vi "LED Lights Subsystem.vi"(8 "error in":errorcluster) -> ()   [LabVIEW 2015]
uses:
  <vilib>/Rock Robotics/SystemInterfaces/i2clib/i2c_bus.ctl
panel:
  in  "Send":bool
  in  "Light ID":u8=3
  in  "Blue":u8=153
  in  "Green":u8=12
  in  "Red":u8=64
  out "error out":errorcluster
  out "open error out":errorcluster
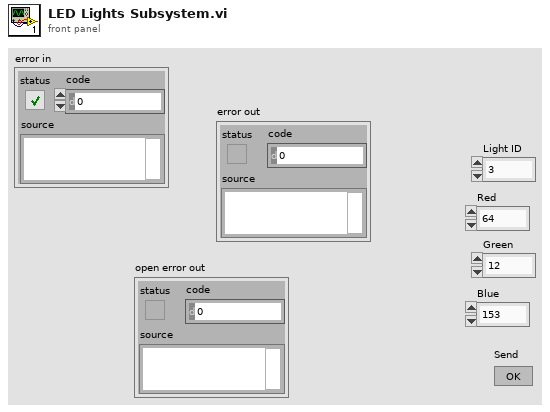
[diagram p1: front panel]
types:
  T1 = typedef "i2c_bus.ctl" = enum16{"I2C On-Board", "I2C MXP", "Invalid"}
  T2 = typedef "WPI_I2CDevRef.ctl" = cluster{"DevStatus":errorcluster, "Device Address":u8, "Handle":i32, "I2C Bus":T1}
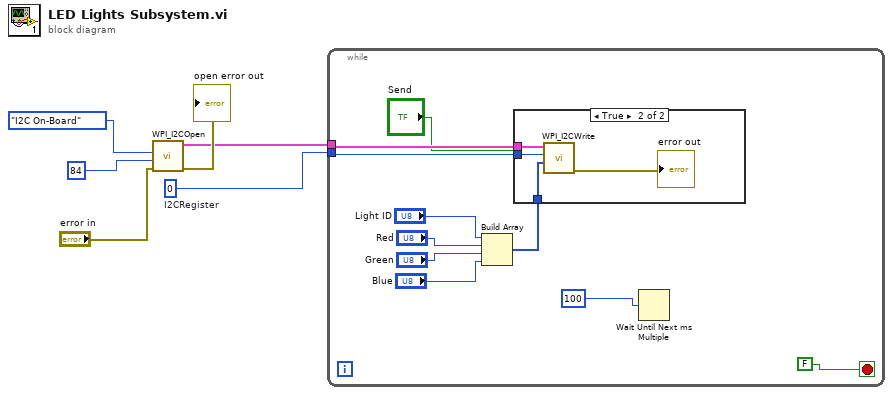
[diagram p0: block diagram]
diagram:
  w1 = u8 0  # I2CRegister
  n1 = call <vilib>:"WPI_I2COpen.vi"("error in"="error in", "Device Address"=u8 84, "I2C Bus"=i2c_bus."I2C On-Board") -> ("error out"=→"open error out":errorcluster, "I2CDevRef"=w2:T2)  [unwired: 7 in]
  n2 = while {
    tunnel: w2 -> [w10]
    tunnel: w1 -> [w9]
    stop <- FALSE stop-if-true
    n3 = Build Array("Light ID", "Red", "Green", "Blue") -> (w15:u8[])
    n4 = case shown="True" "Send" {
      tunnel: w15 -> [_ w20]
      tunnel: w10 -> [_ w19]
      tunnel: w9 -> [_ w18]
      frame False {
      }
      frame True {
        n5 = call <vilib>:"WPI_I2CWrite.vi"("I2CDataToSend"=w20, "I2CRegister"=w18, "I2CDevRef"=w19) -> ("error out"=→"error out":errorcluster)  [unwired: 7 in, 1 out]
      }
    }
    n6 = Wait Until Next ms Multiple(millisecond multiple=100) -> ()  [unwired: 1 out]
  }
